vi "BRig_Host__Loop_Consumer_RunState__getThresholds_v2.vi"(10 "input_idx":i32[](array[numeric]), 11 "input_dataTS":u16[][](array[numeric])) -> (0 "output_threshold_2":u16, 1 "output_threshold_1":u16)   [LabVIEW 2014]
uses:
  <vilib>/Utility/file.llb/Write To Spreadsheet File (DBL).vi
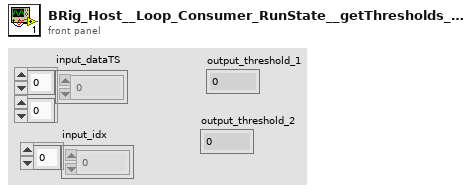
[diagram p1: front panel]
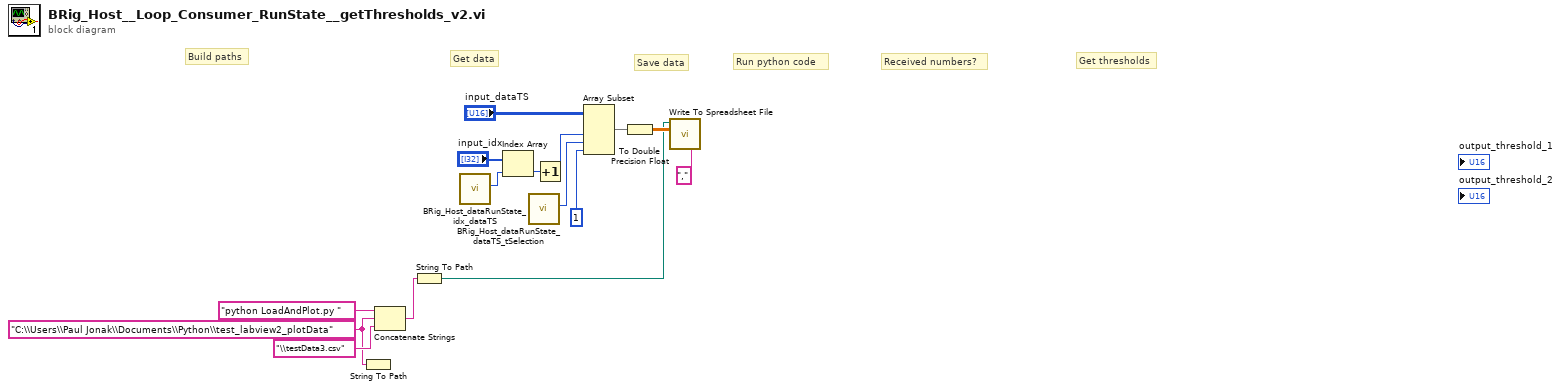
[diagram p0: block diagram]
diagram:
  w13 = "C:\\Users\\Paul Jonak\\Documents\\Python\\test_labview2_plotData"
  # "Get thresholds"
  # "Run python code"
  # "Save data"
  # "Get data"
  # "Build paths"
  # "Received numbers?"
  n1 = String To Path(string=w13) -> ()  [unwired: 1 out]
  n2 = Concatenate Strings("python LoadAndPlot.py " ("command line"), w13, "\\testData3.csv") -> (w2:string)
  n3 = String To Path(string=w2) -> (path=w1:path)
  n4 = call "BRig_Host_dataRunState_idx_dataTS.vi"() -> ("output_idx_dataTS"=w11:i32)  [unwired: 11 in]
  n5 = Index Array(array="input_idx", index=w11) -> (element=w9:i32)
  n6 = call "BRig_Host_dataRunState_dataTS_tSelection.vi"() -> ("output_idx_dataTS_tSelection"=w7:i32)  [unwired: 11 in]
  n7 = Increment(x=w9) -> (x+1=w8:i32)
  n8 = Array Subset(array="input_dataTS", length (row)=w8, index (col)=w7, length (col)=1 ("length")) -> (w5:u16[][])  [unwired: 1 in]
  n9 = To Double Precision Float(number=w5) -> (double precision float=w4:dbl[][])
  n10 = call-poly <vilib>:"Write To Spreadsheet File.vi"("delimiter (\\t)"="," ("delimiter (\\t)"), "2D data"=w4, "file path (dialog if empty)"=w1) -> ()  [unwired: 5 in, 1 out]
